vi "remove multiple dependent node references.vi"(8 "error in (no error)":errorcluster, 10 "Base Property Name":string, 11 "Item Ref in":T1 format="%.0x") -> (0 "error out":errorcluster, 3 "Item Ref out":T1=18446744073709551615 format="%.0x")   [LabVIEW 2016]
uses:
  <vilib>/NI Veristand/Custom Device API/Custom Device Item Ref.ctl
  <vilib>/NI VeriStand/Custom Device API/Custom Device API.lvlib
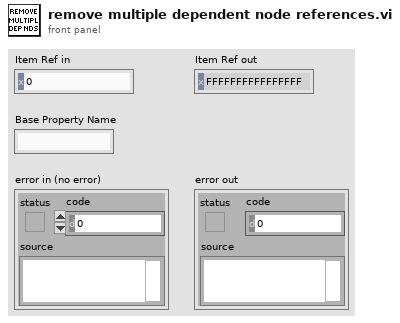
[diagram p1: front panel]
types:
  T1 = typedef "Custom Device API.lvlib/Custom Device Item Ref.ctl" = u64
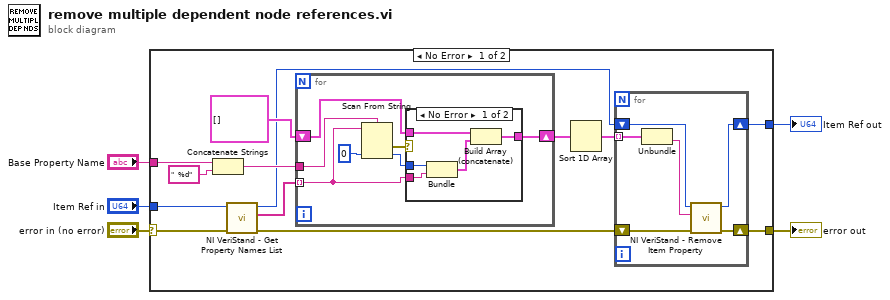
[diagram p0: block diagram]
diagram:
  n1 = case shown="No Error" "error in (no error)" {
    selector: "error in (no error)" -> [w14 w38]
    tunnel: "Item Ref in" -> [w18 w39]
    tunnel: [w9 w39] -> w4
    tunnel: [w8 w38] -> w3
    tunnel: "Base Property Name" -> [w17 _]
    frame No Error {
      n2 = Concatenate Strings(w17, "  %d" ("string")) -> (w15:string)
      n3 = call <vilib>:"NI VeriStand - Get Property Names List.vi"("error in (no error)"=w14, "Item Ref in"=w18) -> ("error out"=w10:errorcluster, "Property Names"=w6:string[], "Item Ref out"=w11:T1)  [unwired: 7 in]
      n4 = for {
        tunnel: w6 -> [w30] mode=indexing
        tunnel: w15 -> [w29]
        shift-right: [w26] -> w12
        shift-left: cluster{"default value 1":i32, string}[] [] -> [w25]
        n5 = Scan From String(format string=w29, input string=w30, default 1=0 ("default value 1")) -> (error out=w31:errorcluster, output 1=w27:i32)  [unwired: 2 in, 2 out]
        n6 = case shown="No Error" w31 {
          tunnel: w30 -> [w35 _]
          tunnel: w27 -> [w36 _]
          tunnel: [w34 w37] -> w26
          tunnel: w25 -> [w33 w37]
          frame No Error {
            n7 = Bundle("default value 1"=w36, w35) -> (w32:cluster{"default value 1":i32, string})  [unwired: 1 in]
            n8 = Build Array (concatenate)(w33, w32) -> (w34:cluster{"default value 1":i32, string}[])
          }
          frame Error {
          }
        }
      }
      n9 = Sort 1D Array(array=w12) -> (sorted array=w7:cluster{"default value 1":i32, string}[])
      n10 = for {
        shift-right: [w22] -> w9
        shift-left: w11 -> [w24]
        shift-right: [w21] -> w8
        shift-left: w10 -> [w23]
        tunnel: w7 -> [w20] mode=indexing
        n11 = Unbundle(w20) -> (w19:string)  [unwired: 1 out]
        n12 = call <vilib>:"NI VeriStand - Remove Item Property.vi"("error in (no error)"=w23, "Property Name"=w19, "Item Ref in"=w24) -> ("error out"=w21:errorcluster, "Item Ref out"=w22:T1)  [unwired: 6 in, 1 out]
      }
    }
    frame Error {
    }
  }
  "Item Ref out" <- w4
  "error out" <- w3
